vi "Process effects.vi"(10 "Apply when":bool, 11 "Effect string":string) -> (3 "Effect":T1[](array[typedef]))   [LabVIEW 2019, in "LSS.lvlib"]
doc: "Takes the effect string and pairs it with the condition when it should be applied.\n\n<b>Inputs:</b>\n<b>Effect string</b> - Line of LSS code that will be applied when the condition is met.\n<b>Apply when</b> - Defines whether this code will be applied when the condition is met, or when it is false.\n<b>Error In</b> - Standard Error In terminal.\n\n<b>Outputs:</b>\n<b>Effect</b> - Effects built as a cluster that will be applied when a certain rules criteria are met.\n<b>Error Out</b> - Standard Error out terminal."
uses:
  LSS.lvlib
  Controls/Effects.ctl
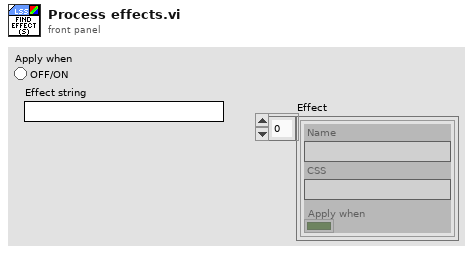
[diagram p1: front panel]
types:
  T1 = typedef "LSS.lvlib/Effects.ctl" = cluster{"Name":string, "CSS":string, "Apply when":bool}
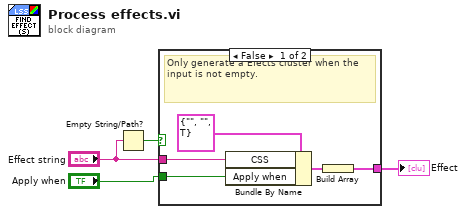
[diagram p0: block diagram]
diagram:
  n1 = Empty String/Path?(string/path="Effect string") -> (empty?=w2:bool)
  n2 = case shown="False" w2 {
    tunnel: "Apply when" -> [w9 _]
    tunnel: "Effect string" -> [w7 _]
    tunnel: [w5 _] -> w3
    frame False {
      # "Only generate a Efects cluster when the input is not empty."
      n3 = Bundle By Name(cluster=T1 {"Name"="", "CSS"="", "Apply when"=TRUE} ("Cluster"), "CSS"=w7, "Apply when"=w9) -> (w6:T1)
      n4 = Build Array(w6) -> (w5:T1[])
    }
    frame True {
    }
  }
  "Effect" <- w3
